vi "getBlockData.vi"(11 "path in":path) -> (2 "Array 2":dbl[](array[numeric]), 3 "Array":dbl[](array[numeric]))   [LabVIEW 2017]
uses:
  <vilib>/Analysis/baseanly.llb/Mean (DBL).vi
  <vilib>/Utility/file.llb/Read Delimited Spreadsheet (DBL).vi
  <vilib>/Analysis/NI_AALBase.lvlib
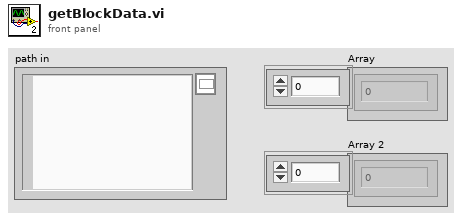
[diagram p1: front panel]
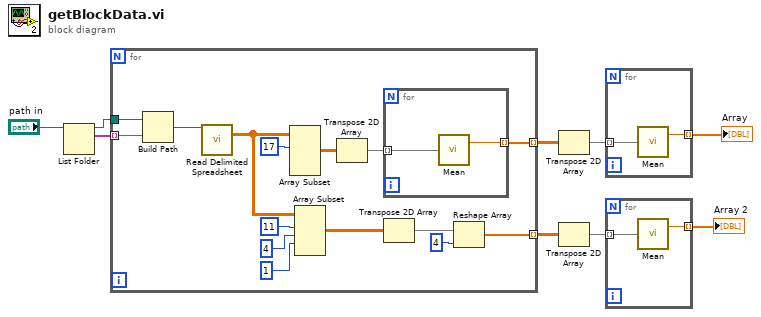
[diagram p0: block diagram]
diagram:
  n1 = List Folder(path="path in") -> (path out=w2:path, filenames=w3:string[])  [unwired: 3 in, 2 out]
  n2 = for {
    tunnel: w2 -> [w24]
    tunnel: w3 -> [w23] mode=indexing
    tunnel: [w17] -> w4 mode=indexing
    tunnel: [w10] -> w7 mode=indexing
    n3 = Build Path(base path=w24, name or relative path=w23) -> (appended path=w22:path)
    n4 = call-poly <vilib>:"Read Delimited Spreadsheet.vi"("file path (dialog if empty)"=w22) -> ("all rows"=w14:dbl[][])  [unwired: 9 in, 5 out]
    n5 = Array Subset(array=w14, index (row)=17 ("index")) -> (w12:dbl[][])  [unwired: 3 in]
    n6 = Array Subset(array=w14, index (row)=11 ("index"), length (row)=4 ("length"), index (col)=1 ("index")) -> (w18:dbl[][])  [unwired: 1 in]
    n7 = Transpose 2D Array(2D array=w12) -> (transposed array=w11:dbl[][])
    n8 = for {
      tunnel: w11 -> [w26] mode=indexing
      tunnel: [w25] -> w10 mode=indexing
      n9 = call-poly <vilib>:"Mean.vi"("X"=w26) -> ("mean"=w25:dbl)  [unwired: 1 out]
    }
    n10 = Transpose 2D Array(2D array=w18) -> (transposed array=w15:dbl[][])
    n11 = Reshape Array(w15, 4 ("dimension size")) -> (w17:dbl[])
  }
  n12 = Transpose 2D Array(2D array=w7) -> (transposed array=w8:dbl[][])
  n13 = Transpose 2D Array(2D array=w4) -> (transposed array=w6:dbl[][])
  n14 = for {
    tunnel: w8 -> [w28] mode=indexing
    tunnel: [w27] -> w9 mode=indexing
    n15 = call-poly <vilib>:"Mean.vi"("X"=w28) -> ("mean"=w27:dbl)  [unwired: 1 out]
  }
  "Array" <- w9
  n16 = for {
    tunnel: w6 -> [w30] mode=indexing
    tunnel: [w29] -> w5 mode=indexing
    n17 = call-poly <vilib>:"Mean.vi"("X"=w30) -> ("mean"=w29:dbl)  [unwired: 1 out]
  }
  "Array 2" <- w5
